vi "RT-MAIN.vi"() -> ()   [LabVIEW 2013]
uses:
  <vilib>/LabVIEW Targets/FPGA/cRIO/shared/nicrio_ModuleControls/nicrio_cRIO-9229_DataRatesRing.ctl
  <vilib>/LabVIEW Targets/FPGA/cRIO/shared/nicrio_ModuleControls/nicrio_cRIO-9205_VoltageRange.ctl
  <vilib>/LabVIEW Targets/FPGA/cRIO/shared/nicrio_ModuleControls/nicrio_cRIO-9205_TerminalMode.ctl
panel:
  out "9205Count(uSec)":u32
  out "9229采样率":u8
  out "9205数据":sgl[](array[numeric])
  out "9229数据":sgl[](array[numeric])
  out "9205fifo flower":bool
  out "9205fifo over":bool
  out "9205剩余元素":u32
  out "9229剩余元素":u32
  out "9229buff overflower":bool
  out "9229buff underflower":bool
  out "9213数据":dbl[](array[numeric])
  out "结果":dbl
  out "结果 2":dbl
  out "元素":string
  out "退出":bool
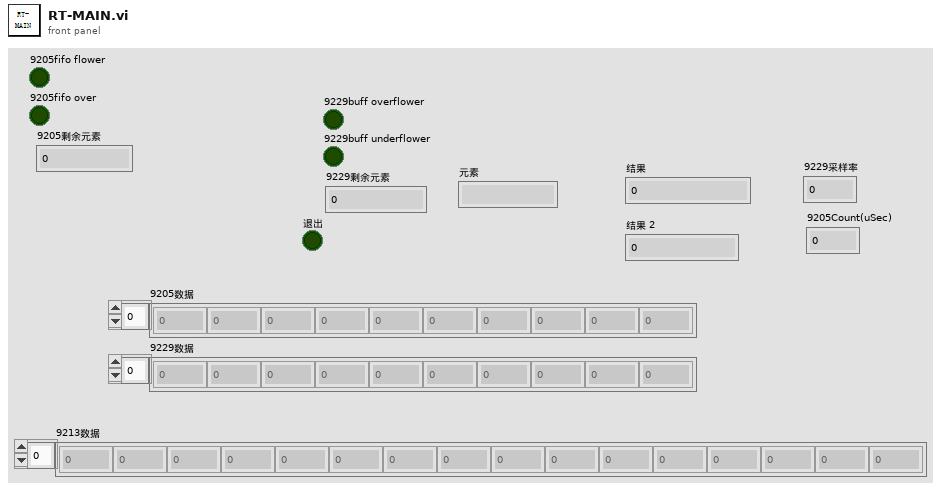
[diagram p1: front panel]
types:
  T1 = typedef "消息命令控件.ctl" = cluster{"message":string, "变体数据":variant}
  T2 = typedef "网络连接枚举控件 .ctl" = enum16{"初始化", "连接UI", "获取UI命令"}
  T3 = typedef "nicrio_cRIO-9229_DataRatesRing.ctl" = u8
  T4 = typedef "nicrio_cRIO-9205_VoltageRange.ctl" = enum8{"+/- 10V", "+/- 5V", "+/- 1V", "+/- 200mV"}
  T5 = typedef "nicrio_cRIO-9205_TerminalMode.ctl" = enum8{"RSE", "NRSE", "DIFF"}
  T6 = cluster{"9205Count(uSec)":u32, "9229采样率":T3, "update9213":bool, "9213转换时间":enum8{"High Speed", "High Resolution"}, "9205Update AI Setings":bool, "9205AI Channel Settings":cluster{"Voltage Range":T4, "Terminal Mode":T5}[]}
  T7 = cluster{"9205Count(uSec)":u32, "9229采样率":u8, "update9213":bool, "9213转换时间":enum8{"High Speed", "High Resolution"}, "9205Update AI Setings":bool, "9205AI Channel Settings":cluster{"Voltage Range":enum8{"+/- 10V", "+/- 5V", "+/- 1V", "+/- 200mV"}, "Terminal Mode":enum8{"RSE", "NRSE", "DIFF"}}[]}
  T8 = cluster{"Voltage Range":enum8{"+/- 10V", "+/- 5V", "+/- 1V", "+/- 200mV"}, "Terminal Mode":enum8{"RSE", "NRSE", "DIFF"}}[]
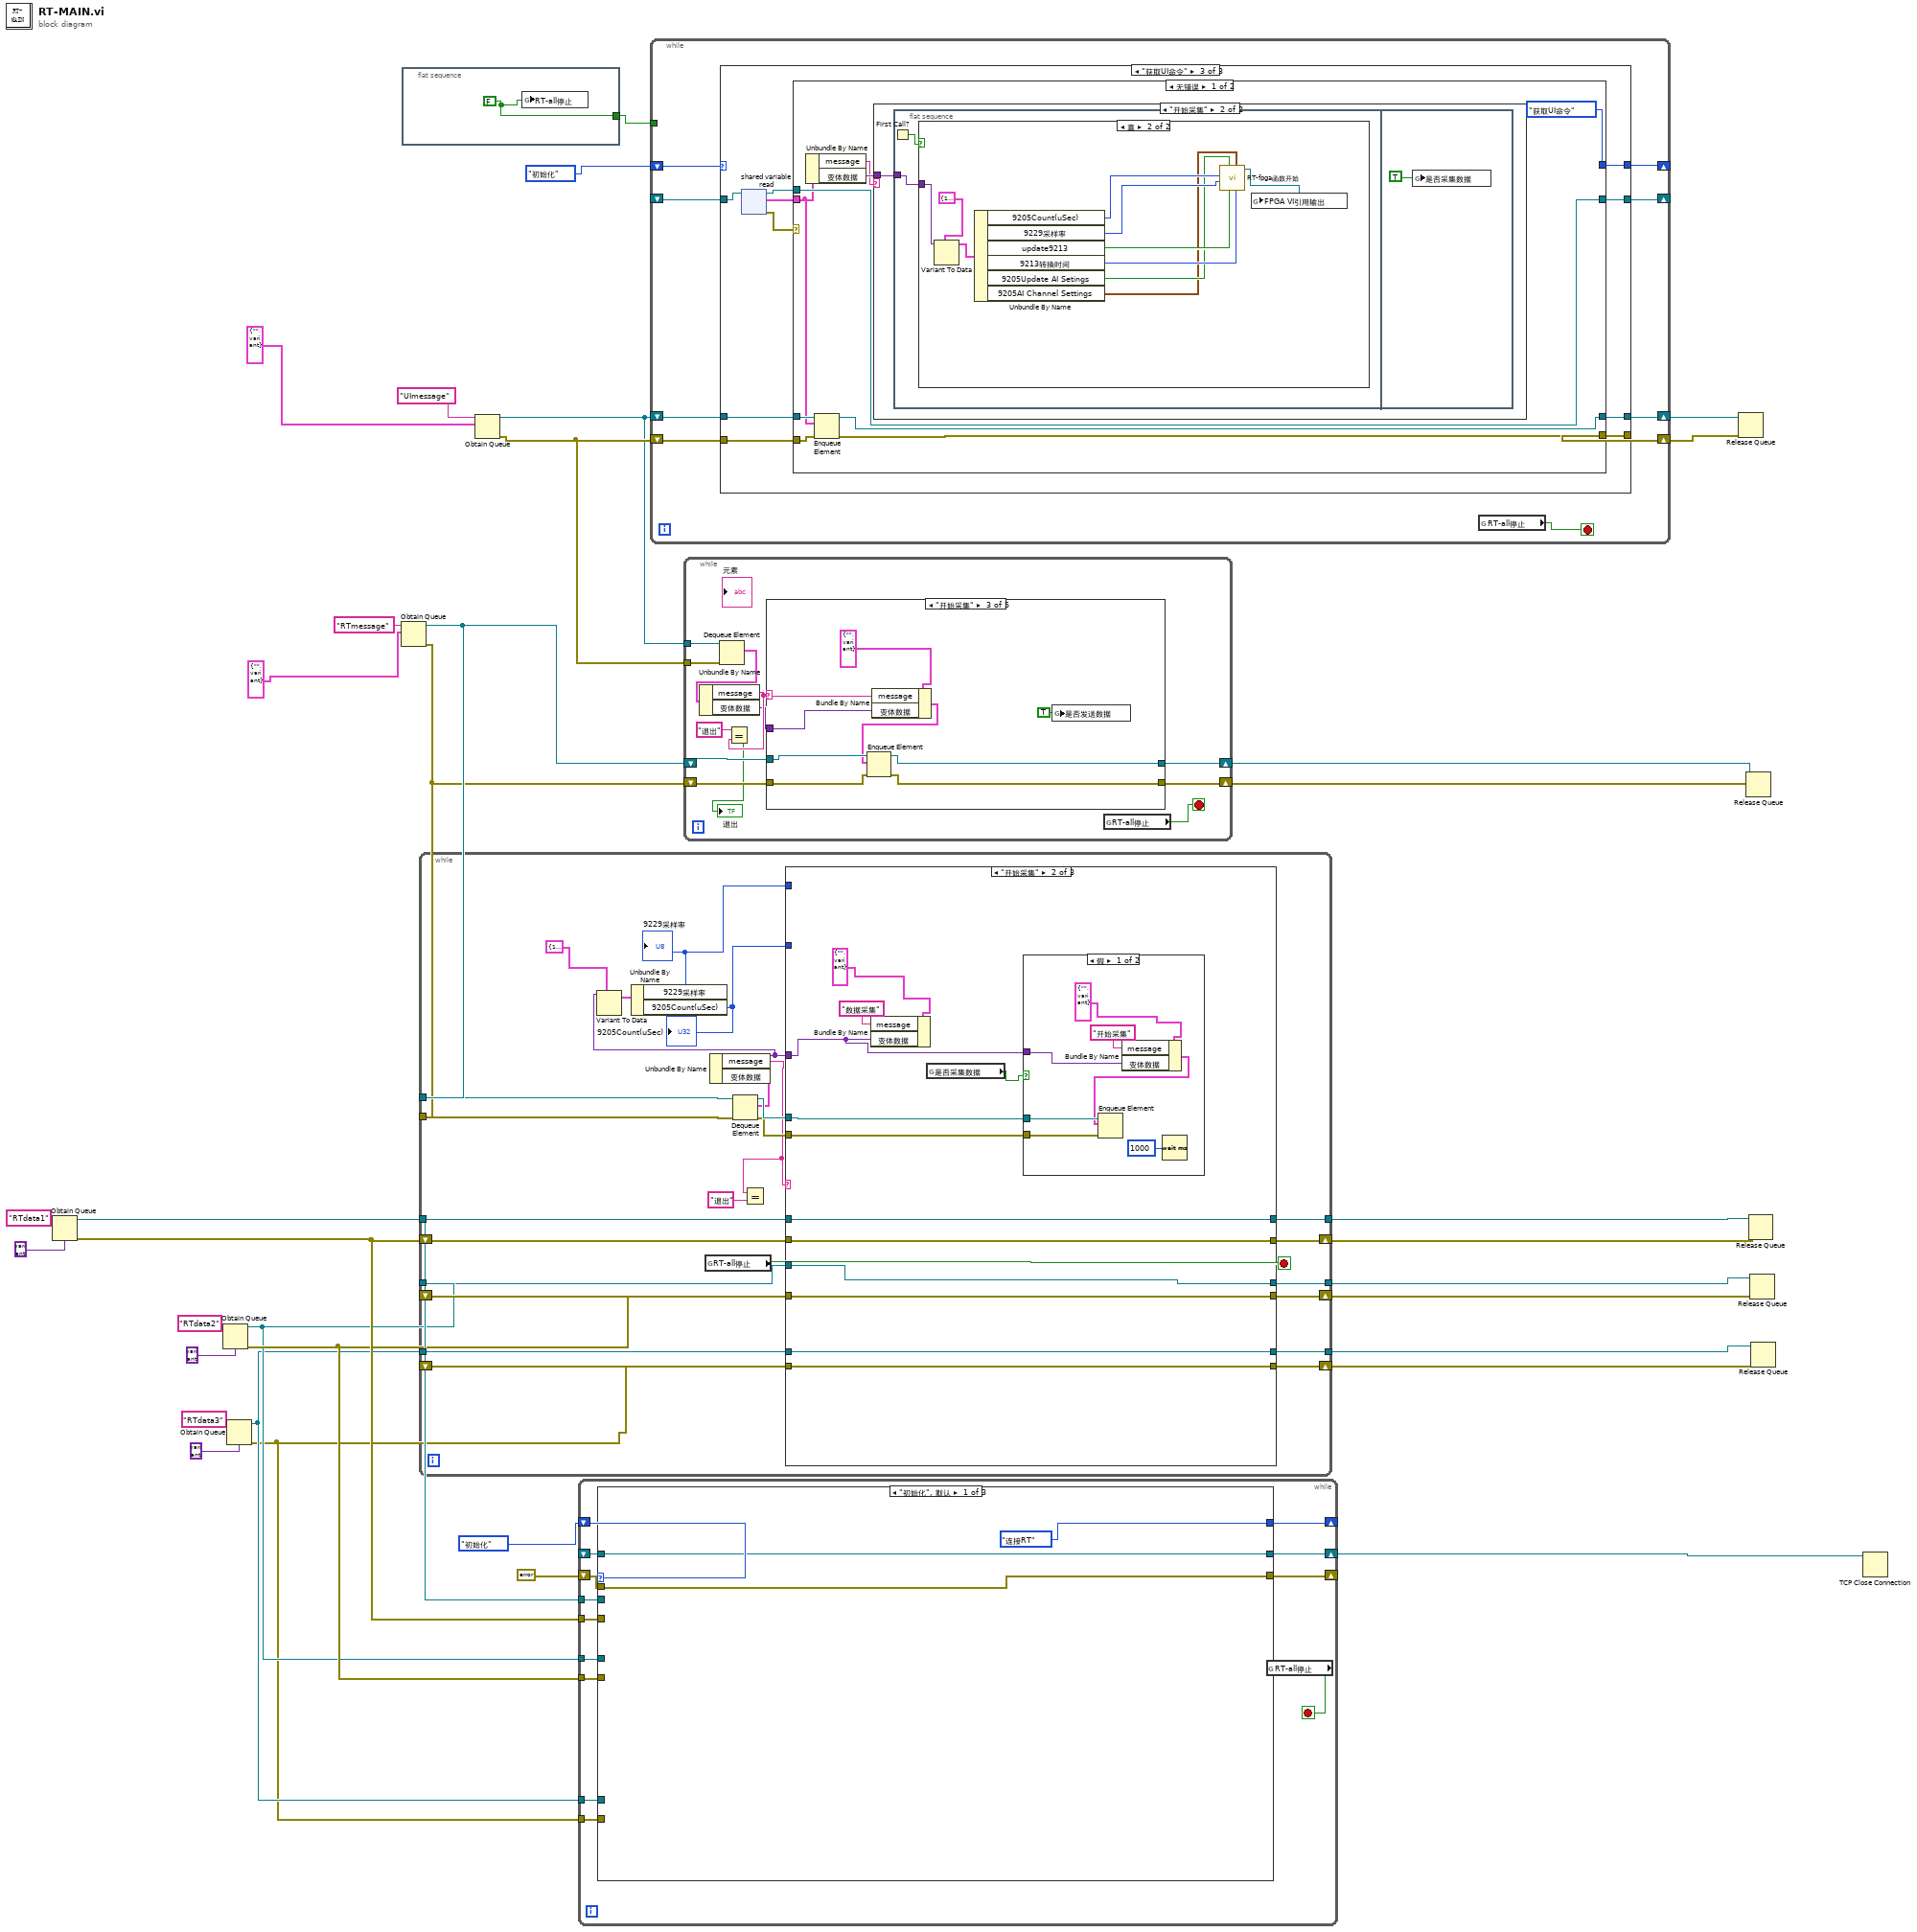
[diagram p0: block diagram]
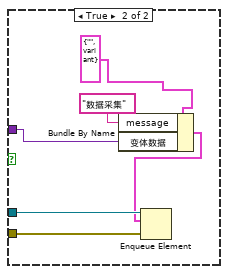
[diagram p3: hidden frame]
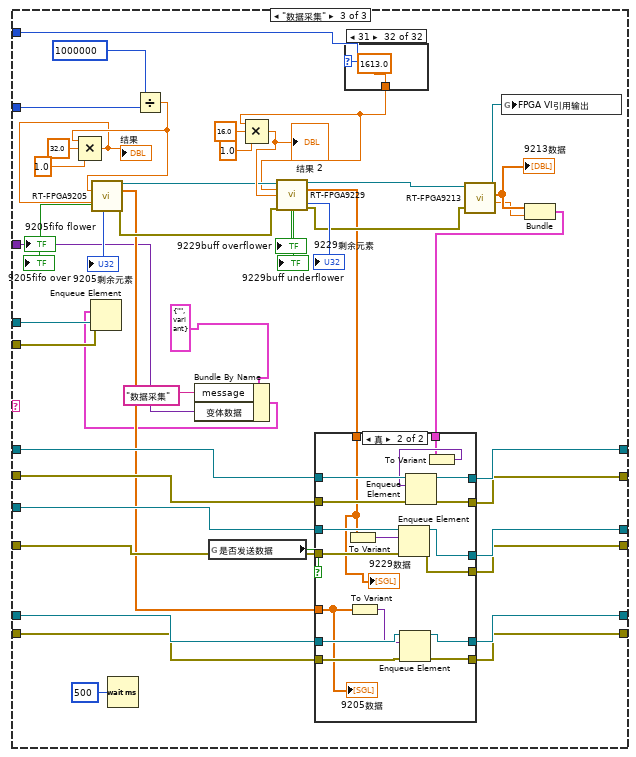
[diagram p4: hidden frame]
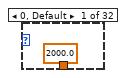
[diagram p5: hidden frame]
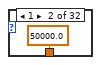
[diagram p6: hidden frame]
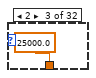
[diagram p7: hidden frame]
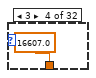
[diagram p8: hidden frame]
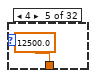
[diagram p9: hidden frame]
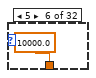
[diagram p10: hidden frame]
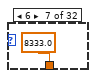
[diagram p11: hidden frame]
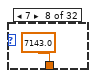
[diagram p12: hidden frame]
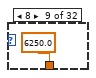
[diagram p13: hidden frame]
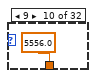
[diagram p14: hidden frame]
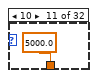
[diagram p15: hidden frame]
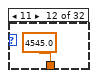
[diagram p16: hidden frame]
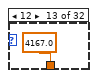
[diagram p17: hidden frame]
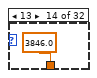
[diagram p18: hidden frame]
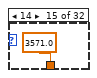
[diagram p19: hidden frame]
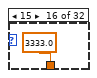
[diagram p20: hidden frame]
diagram:
  n1 = Obtain Queue(name (unnamed)="RTdata1" ("名称（未命名）"), element data type=variant ("变体")) -> (queue out=w23:refnum<queue>, error out=w20:errorcluster)  [unwired: 3 in, 1 out]
  n2 = Obtain Queue(name (unnamed)="RTdata2" ("名称（未命名）"), element data type=variant ("变体")) -> (queue out=w18:refnum<queue>, error out=w19:errorcluster)  [unwired: 3 in, 1 out]
  n3 = Obtain Queue(name (unnamed)="RTdata3" ("名称（未命名）"), element data type=variant ("变体")) -> (queue out=w8:refnum<queue>, error out=w7:errorcluster)  [unwired: 3 in, 1 out]
  n4 = Obtain Queue(name (unnamed)="RTmessage" ("名称（未命名）"), element data type=T1 {"message"="", "变体数据"=variant} ("命令消息")) -> (queue out=w25:refnum<queue>, error out=w24:errorcluster)  [unwired: 3 in, 1 out]
  n5 = flat-sequence {
    tunnel: [w36] -> w11
    frame #0 {
      w36 = FALSE ("停止")
      n6 = global write "RT-all停止全局.vi" "RT-all停止"(w36) -> ()
    }
  }
  n7 = while {
    tunnel: w25 -> [w61]
    tunnel: w24 -> [w60]
    shift-right: [w55] -> w14
    shift-left: w20 -> [w56]
    shift-right: [w51] -> w12
    shift-left: w19 -> [w52]
    shift-right: [w47] -> w5
    shift-left: w7 -> [w49]
    tunnel: w23 -> [w58]
    tunnel: [w57] -> w15
    tunnel: w18 -> [w54]
    tunnel: [w53] -> w13
    tunnel: w8 -> [w50]
    tunnel: [w48] -> w6
    stop <- w42 stop-if-true
    n8 = global read "RT-all停止全局.vi" "RT-all停止"() -> (w42:bool)
    n9 = Dequeue Element(queue=w61, error in (no error)=w60) -> (queue out=w59:refnum<queue>, element=w43:T1, error out=w45:errorcluster)  [unwired: 1 in, 1 out]
    n10 = Unbundle By Name(w43) -> ("message"=w44:string, "变体数据"=w41:variant)
    n11 = Variant To Data(type=T6 {"9205Count(uSec)"=1000, "9229采样率"=25, "update9213"=TRUE, "9213转换时间"=enum."High Speed", "9205Update AI Setings"=TRUE, "9205AI Channel Settings"=[{"Voltage Range"=enum."+/- 10V", "Terminal Mode"=enum."RSE"}, {"Voltage Range"=enum."+/- 10V", "Terminal Mode"=enum."RSE"}, {"Voltage Range"=enum."+/- 10V", "Terminal Mode"=enum."RSE"}, {"Voltage Range"=enum."+/- 10V", "Terminal Mode"=enum."RSE"}, {"Voltage Range"=enum."+/- 10V", "Terminal Mode"=enum."RSE"}, {"Voltage Range"=enum."+/- 10V", "Terminal Mode"=enum."RSE"}, {"Voltage Range"=enum."+/- 10V", "Terminal Mode"=enum."RSE"}, {"Voltage Range"=enum."+/- 10V", "Terminal Mode"=enum."RSE"}, {"Voltage Range"=enum."+/- 10V", "Terminal Mode"=enum."RSE"}, {"Voltage Range"=enum."+/- 10V", "Terminal Mode"=enum."RSE"}, {"Voltage Range"=enum."+/- 10V", "Terminal Mode"=enum."RSE"}, {"Voltage Range"=enum."+/- 10V", "Terminal Mode"=enum."RSE"}, {"Voltage Range"=enum."+/- 10V", "Terminal Mode"=enum."RSE"}, {"Voltage Range"=enum."+/- 10V", "Terminal Mode"=enum."RSE"}, {"Voltage Range"=enum."+/- 10V", "Terminal Mode"=enum."RSE"}, {"Voltage Range"=enum."+/- 10V", "Terminal Mode"=enum."RSE"}, {"Voltage Range"=enum."+/- 10V", "Terminal Mode"=enum."RSE"}, {"Voltage Range"=enum."+/- 10V", "Terminal Mode"=enum."RSE"}, {"Voltage Range"=enum."+/- 10V", "Terminal Mode"=enum."RSE"}, {"Voltage Range"=enum."+/- 10V", "Terminal Mode"=enum."RSE"}, {"Voltage Range"=enum."+/- 10V", "Terminal Mode"=enum."RSE"}, {"Voltage Range"=enum."+/- 10V", "Terminal Mode"=enum."RSE"}, {"Voltage Range"=enum."+/- 10V", "Terminal Mode"=enum."RSE"}, {"Voltage Range"=enum."+/- 10V", "Terminal Mode"=enum."RSE"}, {"Voltage Range"=enum."+/- 10V", "Terminal Mode"=enum."RSE"}]}, Variant=w41) -> (data=w40:T7)  [unwired: 1 in, 1 out]
    n12 = Unbundle By Name(w40) -> ("9229采样率"=w38:u8, "9205Count(uSec)"=w37:u32)
    "9229采样率" <- w38
    "9205Count(uSec)" <- w37
    n13 = Equal?(x=w44, y="退出") -> ()  [unwired: 1 out]
    n14 = case shown="\"开始采集\"" w44 {
      tunnel: w59 -> [_ w71 w139]
      tunnel: w58 -> [w67 w79 w138]
      tunnel: [w67 w79 w137] -> w57
      tunnel: w56 -> [w66 w78 w136]
      tunnel: [w66 w78 w135] -> w55
      tunnel: w54 -> [w65 w77 w134]
      tunnel: [w65 w77 w133] -> w53
      tunnel: w52 -> [w64 w76 w132]
      tunnel: [w64 w76 w131] -> w51
      tunnel: w50 -> [w63 w75 w129]
      tunnel: w49 -> [w62 w74 w128]
      tunnel: [w63 w75 w127] -> w48
      tunnel: [w62 w74 w126] -> w47
      tunnel: w45 -> [_ w70 w125]
      tunnel: w41 -> [_ w69 w110]
      tunnel: w38 -> [_ _ w95]
      tunnel: w37 -> [_ _ w93]
      frame Default {
      }
      frame "开始采集" {
        n15 = Bundle By Name(cluster=T1 {"message"="", "变体数据"=variant} ("命令消息"), "message"="数据采集" ("元素"), "变体数据"=w69) -> ()  [unwired: 1 out]
        n16 = global read "FPGA是否采集全局.vi" "是否采集数据"() -> (w72:bool)
        n17 = case shown="假" w72 {
          tunnel: w71 -> [w84 w92]
          tunnel: w70 -> [w83 w91]
          tunnel: w69 -> [w85 w89]
          frame False {
            n18 = Bundle By Name(cluster=T1 {"message"="", "变体数据"=variant} ("命令消息"), "message"="开始采集" ("元素"), "变体数据"=w85) -> (w82:T1)
            n19 = Enqueue Element(queue=w84, element=w82, error in (no error)=w83) -> ()  [unwired: 1 in, 3 out]
            n20 = Wait (ms)(milliseconds to wait=u32 1000 ("等待时间（毫秒）")) -> ()  [unwired: 1 out]
          }
          frame True {
            n21 = Bundle By Name(cluster=T1 {"message"="", "变体数据"=variant} ("命令消息"), "message"="数据采集" ("元素"), "变体数据"=w89) -> (w88:T1)
            n22 = Enqueue Element(queue=w92, element=w88, error in (no error)=w91) -> ()  [unwired: 1 in, 3 out]
          }
        }
      }
      frame "数据采集" {
        n23 = Wait (ms)(milliseconds to wait=u32 500 ("等待时间（毫秒）")) -> ()  [unwired: 1 out]
        n24 = Divide(x=u32 1000000, y=w93) -> (x/y=w106:dbl)
        n25 = Compound Arithmetic op=MULTIPLY(w106, 32.0 ("值"), 1.0 ("值")) -> (w103:dbl)
        "结果" <- w103
        n26 = call "RT-FPGA9205.vi"("9205采样率"=w106, "9205采样点数"=w103) -> ("FPGA VI引用输出"=w99:refnum<k20>, "9205数据"=w113:sgl[], "9205fifo flower"=→"9205fifo flower":bool, "9205fifo over"=→"9205fifo over":bool, "9205剩余元素"=→"9205剩余元素":u32, "错误输出"=w121:errorcluster)  [unwired: 4 in, 4 out]
        n27 = Bundle By Name(cluster=T1 {"message"="", "变体数据"=variant} ("命令消息"), "message"="数据采集" ("元素"), "变体数据"=w110) -> (w109:T1)
        n28 = Enqueue Element(queue=w139, element=w109, error in (no error)=w125) -> ()  [unwired: 1 in, 3 out]
        n29 = global read "RT是否发送全局.vi" "是否发送数据"() -> (w130:bool)
        n30 = case shown="31" w95 {
          tunnel: [2000.0 ("值") 50000.0 ("值") 25000.0 ("值") 16607.0 ("值") 12500.0 ("值") 10000.0 ("值") 8333.0 ("值") 7143.0 ("值") 6250.0 ("值") 5556.0 ("值") 5000.0 ("值") 4545.0 ("值") 4167.0 ("值") 3846.0 ("值") 3571.0 ("值") 3333.0 ("值") 3125.0 ("值") 2941.0 ("值") 2778.0 ("值") 2632.0 ("值") 2500.0 ("值") 2381.0 ("值") 2273.0 ("值") 2174.0 ("值") 2083.0 ("值") 2000.0 ("值") 1923.0 ("值") 1852.0 ("值") 1786.0 ("值") 1724.0 ("值") 1667.0 ("值") 1613.0 ("值")] -> w94
          frame 0, Default {
          }
          frame 1 {
          }
          frame 2 {
          }
          frame 3 {
          }
          frame 4 {
          }
          frame 5 {
          }
          frame 6 {
          }
          frame 7 {
          }
          frame 8 {
          }
          frame 9 {
          }
          frame 10 {
          }
          frame 11 {
          }
          frame 12 {
          }
          frame 13 {
          }
          frame 14 {
          }
          frame 15 {
          }
          frame 16 {
          }
          frame 17 {
          }
          frame 18 {
          }
          frame 19 {
          }
          frame 20 {
          }
          frame 21 {
          }
          frame 22 {
          }
          frame 23 {
          }
          frame 24 {
          }
          frame 25 {
          }
          frame 26 {
          }
          frame 27 {
          }
          frame 28 {
          }
          frame 29 {
          }
          frame 30 {
          }
          frame 31 {
          }
        }
        n31 = Compound Arithmetic op=MULTIPLY(w94, 16.0 ("值"), 1.0 ("值")) -> (w100:dbl)
        "结果 2" <- w100
        n32 = call "RT-FPGA9229.vi"("FPGA VI引用输入"=w99, "9229采样率"=w94, "9229采样点数"=w100, "错误输入"=w121) -> ("FPGA VI引用输出"=w98:refnum<k20>, "9229数据"=w112:sgl[], "9229剩余元素"=→"9229剩余元素":u32, "9229buff overflower"=→"9229buff overflower":bool, "9229buff underflower"=→"9229buff underflower":bool, "错误输出"=w117:errorcluster)  [unwired: 3 in, 3 out]
        n33 = call "RT-FPGA9213.vi"("错误输入"=w117, "FPGA VI引用输入"=w98) -> ("9213dt 输出"=w114:dbl, "9213输出数组"=w116:dbl[], "FPGA VI引用输出"=w97:refnum<k20>)  [unwired: 4 in, 3 out]
        "9213数据" <- w116
        n34 = global write "RT-FPGA引用全局.vi" "FPGA VI引用输出"(w97) -> ()
        n35 = Bundle("9213输出数组"=w116, "9213dt 输出"=w114) -> (w115:cluster{"9213输出数组":dbl[], "9213dt 输出":dbl})  [unwired: 1 in]
        n36 = case shown="真" w130 {
          tunnel: w138 -> [w177 w195]
          tunnel: [w177 w194] -> w137
          tunnel: w136 -> [w176 w193]
          tunnel: [w176 w192] -> w135
          tunnel: w134 -> [w175 w191]
          tunnel: [w175 w190] -> w133
          tunnel: w132 -> [w174 w189]
          tunnel: [w174 w188] -> w131
          tunnel: w129 -> [w173 w186]
          tunnel: w128 -> [w172 w185]
          tunnel: [w173 w184] -> w127
          tunnel: [w172 w183] -> w126
          tunnel: w115 -> [_ w180]
          tunnel: w113 -> [_ w179]
          tunnel: w112 -> [_ w178]
          frame False {
          }
          frame True {
            n37 = To Variant(anything=w178) -> (Variant=w187:variant)
            n38 = To Variant(anything=w179) -> (Variant=w182:variant)
            n39 = Enqueue Element(queue=w191, element=w187, error in (no error)=w189) -> (queue out=w190:refnum<queue>, error out=w188:errorcluster)  [unwired: 1 in, 1 out]
            n40 = Enqueue Element(queue=w186, element=w182, error in (no error)=w185) -> (queue out=w184:refnum<queue>, error out=w183:errorcluster)  [unwired: 1 in, 1 out]
            n41 = To Variant(anything=w180) -> (Variant=w181:variant)
            n42 = Enqueue Element(queue=w195, element=w181, error in (no error)=w193) -> (queue out=w194:refnum<queue>, error out=w192:errorcluster)  [unwired: 1 in, 1 out]
            "9205数据" <- w179
            "9229数据" <- w178
          }
        }
      }
    }
  }
  n43 = Obtain Queue(name (unnamed)="UImessage" ("名称（未命名）"), element data type=T1 {"message"="", "变体数据"=variant} ("命令消息")) -> (queue out=w30:refnum<queue>, error out=w31:errorcluster)  [unwired: 3 in, 1 out]
  n44 = while {
    shift-right: [w207] -> _
    shift-left: enum16{"初始化", "连接RT", "开始传输"}."初始化" -> [w208]
    shift-right: [w206] -> w27
    shift-left: _ -> [w205]
    tunnel: w23 -> [w204]
    tunnel: w20 -> [w202]
    tunnel: w19 -> [w201]
    tunnel: w18 -> [w200]
    tunnel: w8 -> [w199]
    tunnel: w7 -> [w198]
    shift-right: [w197] -> _
    shift-left: errorcluster {"status"=FALSE, "code"=0, "source"=""} ("error IO") -> [w196]
    stop <- w203 stop-if-true
    n45 = case shown="\"初始化\", 默认" w208 {
      tunnel: [enum16{"初始化", "连接RT", "开始传输"}."连接RT" w222 w274] -> w207
      tunnel: [w210 w212 w272] -> w206
      tunnel: w205 -> [w210 w213 _]
      tunnel: w204 -> [_ w236 _]
      tunnel: w202 -> [_ w235 _]
      tunnel: w201 -> [_ w234 _]
      tunnel: w200 -> [_ w233 _]
      tunnel: w199 -> [_ w227 _]
      tunnel: w198 -> [_ w226 _]
      tunnel: [w209 w216 w270] -> w197
      tunnel: w196 -> [w209 w215 _]
      frame "初始化", Default {
      }
      frame "开始传输" {
        n46 = case shown="无错误" w215 {
          tunnel: [w265 _] -> w239
          tunnel: [w264 _] -> w237
          tunnel: w236 -> [w263 _]
          tunnel: w235 -> [w260 _]
          tunnel: w234 -> [w259 _]
          tunnel: w233 -> [w258 _]
          tunnel: [w254 _] -> w231
          tunnel: [w253 _] -> w230
          tunnel: w227 -> [w250 _]
          tunnel: w226 -> [w249 _]
          tunnel: [w247 _] -> w225
          tunnel: [w245 _] -> w224
          tunnel: [enum16{"初始化", "连接RT", "开始传输"}."开始传输" enum16{"初始化", "连接RT", "开始传输"}."连接RT"] -> w222
          tunnel: [w240 refnum<k5> refnum ("connection ID")] -> w214
          tunnel: w213 -> [w240 w267]
          frame No Error {
            n47 = Dequeue Element(queue=w250, error in (no error)=w249) -> (element=w248:variant)  [unwired: 1 in, 3 out]
            n48 = Dequeue Element(queue=w263, error in (no error)=w260) -> (element=w262:variant)  [unwired: 1 in, 3 out]
            n49 = Dequeue Element(queue=w258, error in (no error)=w259) -> (element=w257:variant)  [unwired: 1 in, 3 out]
            n50 = Variant To Data(type=cluster{"9213输出数组":dbl[], "9213dt 输出":dbl} {"9213输出数组"=[], "9213dt 输出"=0.0} ("输出簇"), Variant=w262) -> (data=w242:cluster{"9213输出数组":dbl[], "9213dt 输出":dbl})  [unwired: 1 in, 1 out]
            n51 = Unbundle(w242) -> ("9213输出数组"=w244:dbl[])  [unwired: 1 out]
            n52 = Type Cast(x=w244) -> (*(type *) &x=w264:string)  [unwired: 1 in]
            n53 = String Length(string=w264) -> (length=w266:i32)
            n54 = Type Cast(x=w266) -> (*(type *) &x=w265:string)  [unwired: 1 in]
            n55 = Variant To Data(type=dbl[] [], Variant=w257) -> (data=w255:dbl[])  [unwired: 1 in, 1 out]
            n56 = Type Cast(x=w255) -> (*(type *) &x=w253:string)  [unwired: 1 in]
            n57 = String Length(string=w253) -> (length=w261:i32)
            n58 = Type Cast(x=w261) -> (*(type *) &x=w254:string)  [unwired: 1 in]
            n59 = Variant To Data(type=dbl[] [], Variant=w248) -> (data=w246:dbl[])  [unwired: 1 in, 1 out]
            n60 = Type Cast(x=w246) -> (*(type *) &x=w245:string)  [unwired: 1 in]
            n61 = String Length(string=w245) -> (length=w251:i32)
            n62 = Type Cast(x=w251) -> (*(type *) &x=w247:string)  [unwired: 1 in]
          }
          frame Error {
            n63 = TCP Close Connection(connection ID=w267) -> ()  [unwired: 2 in, 2 out]
          }
        }
        n64 = TCP Write(connection ID=w214, data in=w239, error in (no error)=w215) -> (connection ID out=w238:refnum<k5>, error out=w221:errorcluster)  [unwired: 1 in, 1 out]
        n65 = TCP Write(connection ID=w238, data in=w237, error in (no error)=w221) -> (connection ID out=w223:refnum<k5>, error out=w220:errorcluster)  [unwired: 1 in, 1 out]
        n66 = TCP Write(connection ID=w223, data in=w231, error in (no error)=w220) -> (connection ID out=w232:refnum<k5>, error out=w219:errorcluster)  [unwired: 1 in, 1 out]
        n67 = TCP Write(connection ID=w232, data in=w230, error in (no error)=w219) -> (connection ID out=w229:refnum<k5>, error out=w218:errorcluster)  [unwired: 1 in, 1 out]
        n68 = TCP Write(connection ID=w229, data in=w225, error in (no error)=w218) -> (connection ID out=w228:refnum<k5>, error out=w217:errorcluster)  [unwired: 1 in, 1 out]
        n69 = TCP Write(connection ID=w228, data in=w224, error in (no error)=w217) -> (connection ID out=w212:refnum<k5>, error out=w216:errorcluster)  [unwired: 1 in, 1 out]
      }
      frame "连接RT" {
        n70 = call <vilib>:"TCP Listen.vi"("port"=u16 6001, "service name"="169.254.66.16") -> ("error out"=w273:errorcluster, "connection ID"=w271:refnum<k5>)  [unwired: 5 in, 3 out]
        n71 = case shown="无错误" w273 {
          selector: w273 -> [w277 w280]
          tunnel: [enum16{"初始化", "连接RT", "开始传输"}."开始传输" enum16{"初始化", "连接RT", "开始传输"}."连接RT"] -> w274
          tunnel: [w278 refnum<k5> refnum ("connection ID")] -> w272
          tunnel: w271 -> [w278 w282]
          tunnel: [w277 w280] -> w270
          frame No Error {
          }
          frame Error {
            n72 = TCP Close Connection(connection ID=w282) -> ()  [unwired: 2 in, 2 out]
          }
        }
      }
    }
    n73 = global read "RT-all停止全局.vi" "RT-all停止"() -> (w203:bool)
  }
  n74 = while {
    shift-right: [w291] -> w33
    shift-left: w30 -> [w292]
    shift-right: [w289] -> w32
    shift-left: w31 -> [w290]
    tunnel: w11 -> [_]
    shift-right: [w287] -> _
    shift-left: 网络连接枚举控件_."初始化" ("网络连接枚举控件") -> [w288]
    shift-right: [w285] -> _
    shift-left: _ -> [w284]
    stop <- w286 stop-if-true
    n75 = case shown="\"获取UI命令\"" w288 {
      tunnel: w292 -> [w296 w306 w321]
      tunnel: [w296 w306 w320] -> w291
      tunnel: [w295 w305 w319] -> w289
      tunnel: w290 -> [w295 w305 w318]
      tunnel: [网络连接枚举控件_."连接UI" ("网络连接枚举控件") w298 w314] -> w287
      tunnel: [w293 w297 w313] -> w285
      tunnel: w284 -> [w293 _ w312]
      frame "初始化", Default {
      }
      frame "连接UI" {
        n76 = Create Network Stream Reader Endpoint(7:50000 ("写入方缓冲大小"), 9:T1 {"message"="", "变体数据"=variant} ("命令消息"), 10:"//169.254.66.16/UI" ("读取方url"), 11:"RT" ("写入方名称")) -> (0:w300:errorcluster, 3:w299:refnum<k21>)  [unwired: 3 in]
        n77 = case shown="错误" w300 {
          tunnel: [网络连接枚举控件_."获取UI命令" ("网络连接枚举控件") 网络连接枚举控件_."连接UI" ("网络连接枚举控件")] -> w298
          tunnel: [w308 refnum<k21> refnum ("写入方名称")] -> w297
          tunnel: w299 -> [w308 w311]
          frame No Error {
          }
          frame Error {
            n78 = Destroy Stream Endpoint(11:w311) -> ()  [unwired: 1 in, 1 out]
          }
        }
      }
      frame "获取UI命令" {
        n79 = shared-variable-read(w312) -> (w315:refnum<k21>, w316:errorcluster, w317:T1)  [unwired: 2 in, 1 out]
        n80 = case shown="无错误" w316 {
          tunnel: w321 -> [w330 w361]
          tunnel: [w329 w361] -> w320
          tunnel: [w328 w360] -> w319
          tunnel: w318 -> [w327 w360]
          tunnel: w317 -> [w323 _]
          tunnel: w315 -> [w324 w359]
          tunnel: [网络连接枚举控件_."获取UI命令" ("网络连接枚举控件") 网络连接枚举控件_."连接UI" ("网络连接枚举控件")] -> w314
          tunnel: [w324 refnum<k21> refnum ("写入方名称")] -> w313
          frame No Error {
            n81 = Unbundle By Name(w323) -> ("message"=w322:string, "变体数据"=w326:variant)
            n82 = Enqueue Element(queue=w330, element=w323, error in (no error)=w327) -> (queue out=w329:refnum<queue>, error out=w328:errorcluster)  [unwired: 1 in, 1 out]
            n83 = case shown="\"开始采集\"" w322 {
              tunnel: w326 -> [_ w331]
              frame "假", Default {
              }
              frame "开始采集" {
                n84 = flat-sequence {
                  tunnel: w331 -> [w332]
                  frame #0 {
                    n85 = First Call?() -> (First Call?: T/F=w333:bool)
                    n86 = case shown="真" w333 {
                      tunnel: w332 -> [w334 w345]
                      frame False {
                        n87 = Variant To Data(type=T6 {"9205Count(uSec)"=1000, "9229采样率"=25, "update9213"=TRUE, "9213转换时间"=enum."High Speed", "9205Update AI Setings"=TRUE, "9205AI Channel Settings"=[{"Voltage Range"=enum."+/- 10V", "Terminal Mode"=enum."RSE"}, {"Voltage Range"=enum."+/- 10V", "Terminal Mode"=enum."RSE"}, {"Voltage Range"=enum."+/- 10V", "Terminal Mode"=enum."RSE"}, {"Voltage Range"=enum."+/- 10V", "Terminal Mode"=enum."RSE"}, {"Voltage Range"=enum."+/- 10V", "Terminal Mode"=enum."RSE"}, {"Voltage Range"=enum."+/- 10V", "Terminal Mode"=enum."RSE"}, {"Voltage Range"=enum."+/- 10V", "Terminal Mode"=enum."RSE"}, {"Voltage Range"=enum."+/- 10V", "Terminal Mode"=enum."RSE"}, {"Voltage Range"=enum."+/- 10V", "Terminal Mode"=enum."RSE"}, {"Voltage Range"=enum."+/- 10V", "Terminal Mode"=enum."RSE"}, {"Voltage Range"=enum."+/- 10V", "Terminal Mode"=enum."RSE"}, {"Voltage Range"=enum."+/- 10V", "Terminal Mode"=enum."RSE"}, {"Voltage Range"=enum."+/- 10V", "Terminal Mode"=enum."RSE"}, {"Voltage Range"=enum."+/- 10V", "Terminal Mode"=enum."RSE"}, {"Voltage Range"=enum."+/- 10V", "Terminal Mode"=enum."RSE"}, {"Voltage Range"=enum."+/- 10V", "Terminal Mode"=enum."RSE"}, {"Voltage Range"=enum."+/- 10V", "Terminal Mode"=enum."RSE"}, {"Voltage Range"=enum."+/- 10V", "Terminal Mode"=enum."RSE"}, {"Voltage Range"=enum."+/- 10V", "Terminal Mode"=enum."RSE"}, {"Voltage Range"=enum."+/- 10V", "Terminal Mode"=enum."RSE"}, {"Voltage Range"=enum."+/- 10V", "Terminal Mode"=enum."RSE"}, {"Voltage Range"=enum."+/- 10V", "Terminal Mode"=enum."RSE"}, {"Voltage Range"=enum."+/- 10V", "Terminal Mode"=enum."RSE"}, {"Voltage Range"=enum."+/- 10V", "Terminal Mode"=enum."RSE"}, {"Voltage Range"=enum."+/- 10V", "Terminal Mode"=enum."RSE"}]}, Variant=w334) -> (data=w342:T7)  [unwired: 1 in, 1 out]
                        n88 = Unbundle By Name(w342) -> ("9205Count(uSec)"=w341:u32, "9229采样率"=w340:u8, "update9213"=w339:bool, "9213转换时间"=w338:enum8{"High Speed", "High Resolution"}, "9205Update AI Setings"=w337:bool, "9205AI Channel Settings"=w336:T8)
                        n89 = call "RT-FPGA函数重置.vi"("9213转换时间"=w338, "9205AI Channel Settings"=w336, "update9213"=w339, "9205Update AI Setings"=w337, "9229采样率"=w340, "9205Count(uSec)"=w341) -> ("FPGA VI引用输出"=w335:refnum<k20>)  [unwired: 4 in, 1 out]
                        n90 = global write "RT-FPGA引用全局.vi" "FPGA VI引用输出"(w335) -> ()
                      }
                      frame True {
                        n91 = Variant To Data(type=T6 {"9205Count(uSec)"=1000, "9229采样率"=25, "update9213"=TRUE, "9213转换时间"=enum."High Speed", "9205Update AI Setings"=TRUE, "9205AI Channel Settings"=[{"Voltage Range"=enum."+/- 10V", "Terminal Mode"=enum."RSE"}, {"Voltage Range"=enum."+/- 10V", "Terminal Mode"=enum."RSE"}, {"Voltage Range"=enum."+/- 10V", "Terminal Mode"=enum."RSE"}, {"Voltage Range"=enum."+/- 10V", "Terminal Mode"=enum."RSE"}, {"Voltage Range"=enum."+/- 10V", "Terminal Mode"=enum."RSE"}, {"Voltage Range"=enum."+/- 10V", "Terminal Mode"=enum."RSE"}, {"Voltage Range"=enum."+/- 10V", "Terminal Mode"=enum."RSE"}, {"Voltage Range"=enum."+/- 10V", "Terminal Mode"=enum."RSE"}, {"Voltage Range"=enum."+/- 10V", "Terminal Mode"=enum."RSE"}, {"Voltage Range"=enum."+/- 10V", "Terminal Mode"=enum."RSE"}, {"Voltage Range"=enum."+/- 10V", "Terminal Mode"=enum."RSE"}, {"Voltage Range"=enum."+/- 10V", "Terminal Mode"=enum."RSE"}, {"Voltage Range"=enum."+/- 10V", "Terminal Mode"=enum."RSE"}, {"Voltage Range"=enum."+/- 10V", "Terminal Mode"=enum."RSE"}, {"Voltage Range"=enum."+/- 10V", "Terminal Mode"=enum."RSE"}, {"Voltage Range"=enum."+/- 10V", "Terminal Mode"=enum."RSE"}, {"Voltage Range"=enum."+/- 10V", "Terminal Mode"=enum."RSE"}, {"Voltage Range"=enum."+/- 10V", "Terminal Mode"=enum."RSE"}, {"Voltage Range"=enum."+/- 10V", "Terminal Mode"=enum."RSE"}, {"Voltage Range"=enum."+/- 10V", "Terminal Mode"=enum."RSE"}, {"Voltage Range"=enum."+/- 10V", "Terminal Mode"=enum."RSE"}, {"Voltage Range"=enum."+/- 10V", "Terminal Mode"=enum."RSE"}, {"Voltage Range"=enum."+/- 10V", "Terminal Mode"=enum."RSE"}, {"Voltage Range"=enum."+/- 10V", "Terminal Mode"=enum."RSE"}, {"Voltage Range"=enum."+/- 10V", "Terminal Mode"=enum."RSE"}]}, Variant=w345) -> (data=w353:T7)  [unwired: 1 in, 1 out]
                        n92 = Unbundle By Name(w353) -> ("9205Count(uSec)"=w352:u32, "9229采样率"=w351:u8, "update9213"=w350:bool, "9213转换时间"=w349:enum8{"High Speed", "High Resolution"}, "9205Update AI Setings"=w348:bool, "9205AI Channel Settings"=w347:T8)
                        n93 = call "RT-fpga函数开始.vi"("9213转换时间"=w349, "9205AI Channel Settings"=w347, "update9213"=w350, "9205Update AI Setings"=w348, "9229采样率"=w351, "9205Count(uSec)"=w352) -> ("FPGA VI引用输出"=w346:refnum<k20>)  [unwired: 4 in, 1 out]
                        n94 = global write "RT-FPGA引用全局.vi" "FPGA VI引用输出"(w346) -> ()
                      }
                    }
                  }
                  frame #1 {
                    n95 = global write "FPGA是否采集全局.vi" "是否采集数据"(TRUE ("采集数据？")) -> ()
                  }
                }
              }
            }
          }
          frame Error {
            n96 = Destroy Stream Endpoint(11:w359) -> ()  [unwired: 1 in, 1 out]
            n97 = global write "FPGA是否采集全局.vi" "是否采集数据"(FALSE ("采集数据？")) -> ()
            n98 = global write "RT是否发送全局.vi" "是否发送数据"(FALSE ("是否采集？")) -> ()
          }
        }
      }
    }
    n99 = global read "RT-all停止全局.vi" "RT-all停止"() -> (w286:bool)
  }
  n100 = while {
    tunnel: w30 -> [w372]
    tunnel: w31 -> [w373]
    shift-right: [w370] -> w17
    shift-left: w25 -> [w371]
    shift-right: [w368] -> w16
    shift-left: w24 -> [w369]
    stop <- w367 stop-if-true
    n101 = Dequeue Element(queue=w372, error in (no error)=w373) -> (element=w366:T1)  [unwired: 1 in, 3 out]
    n102 = Unbundle By Name(w366) -> ("message"=w365:string, "变体数据"=w363:variant)
    n103 = Equal?(x="退出" ("y"), y=w365) -> (x = y?=→"退出":bool)
    n104 = case shown="\"开始采集\"" w365 {
      selector: w365 -> [_ _ w380 _ w394]
      tunnel: w371 -> [w375 w378 w387 w390 w399]
      tunnel: [w375 w378 w386 w390 w397] -> w370
      tunnel: w369 -> [w374 w377 w385 w389 w398]
      tunnel: [w374 w377 w384 w389 w396] -> w368
      tunnel: w363 -> [_ _ w382 _ w395]
      frame "初始化" {
        n105 = global write "RT是否发送全局.vi" "是否发送数据"(TRUE ("布尔")) -> ()
      }
      frame Default {
      }
      frame "开始采集" {
        n106 = Bundle By Name(cluster=T1 {"message"="", "变体数据"=variant} ("命令消息"), "message"=w380, "变体数据"=w382) -> (w381:T1)
        n107 = Enqueue Element(queue=w387, element=w381, error in (no error)=w385) -> (queue out=w386:refnum<queue>, error out=w384:errorcluster)  [unwired: 1 in, 1 out]
        n108 = global write "RT是否发送全局.vi" "是否发送数据"(TRUE ("是否采集？")) -> ()
      }
      frame "停止采集" {
        n109 = global write "RT是否发送全局.vi" "是否发送数据"(FALSE ("布尔")) -> ()
      }
      frame "退出" {
        n110 = Bundle By Name(cluster=T1 {"message"="", "变体数据"=variant} ("命令消息"), "message"=w394, "变体数据"=w395) -> (w393:T1)
        n111 = Enqueue Element(queue=w399, element=w393, error in (no error)=w398) -> (queue out=w397:refnum<queue>, error out=w396:errorcluster)  [unwired: 1 in, 1 out]
        n112 = global write "RT是否发送全局.vi" "是否发送数据"(FALSE ("是否采集？")) -> ()
      }
    }
    n113 = global read "RT-all停止全局.vi" "RT-all停止"() -> (w367:bool)
  }
  n114 = Release Queue(queue=w33, error in (no error)=w32) -> ()  [unwired: 1 in, 3 out]
  n115 = Release Queue(queue=w17, error in (no error)=w16) -> ()  [unwired: 1 in, 3 out]
  n116 = Release Queue(queue=w15, error in (no error)=w14) -> ()  [unwired: 1 in, 3 out]
  n117 = Release Queue(queue=w13, error in (no error)=w12) -> ()  [unwired: 1 in, 3 out]
  n118 = Release Queue(queue=w6, error in (no error)=w5) -> ()  [unwired: 1 in, 3 out]
  n119 = TCP Close Connection(connection ID=w27) -> ()  [unwired: 2 in, 2 out]
